vi "ma_sml_Default Center and Span.vi"(0 "fs":dbl=1024.0 format="%.2f", 1 "effective band specification":cluster{"fl (vs. fs)":dbl, "fh (vs. fs)":dbl}={"fl (vs. fs)"=0.0, "fh (vs. fs)"=0.5} {"fh (vs. fs)" format="%.2f"; "fl (vs. fs)" format="%.2f"}, 2 "input signal type":enum16{"real", "complex modulated"}(ring)) -> (3 "f center":dbl=1024.0 format="%.2f", 4 "f upper":dbl=1024.0 format="%.2f", 5 "f lower":dbl=1024.0 format="%.2f", 6 "max span":dbl=1024.0 format="%.2f")   [LabVIEW 2020, in "NI_MAPro.lvlib"]
uses:
  NI_MAPro.lvlib
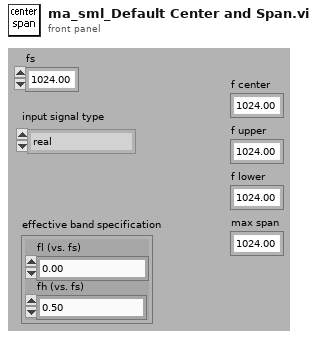
[diagram p1: front panel]
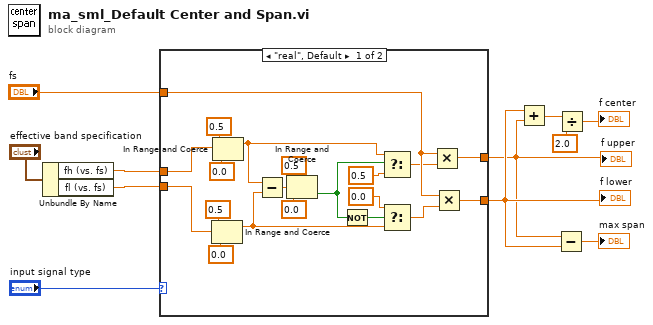
[diagram p0: block diagram]
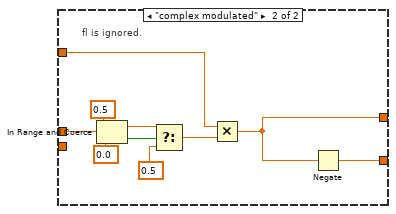
[diagram p2: hidden frame]
diagram:
  n1 = Unbundle By Name("effective band specification") -> ("fh (vs. fs)"=w4:dbl, "fl (vs. fs)"=w5:dbl)
  n2 = case shown="\"real\", Default" "input signal type" {
    tunnel: "fs" -> [w31 w32]
    tunnel: [w30 w34] -> w8
    tunnel: [w29 w33] -> w7
    tunnel: w5 -> [w28 _]
    tunnel: w4 -> [w27 w39]
    frame "real", Default {
      n3 = In Range and Coerce(upper limit=0.5, x=w28, lower limit=0.0) -> (coerced(x)=w16:dbl)  [unwired: 1 out]
      n4 = In Range and Coerce(upper limit=0.5, x=w27, lower limit=0.0) -> (coerced(x)=w19:dbl)  [unwired: 1 out]
      n5 = Subtract(x=w19, y=w16) -> (x-y=w22:dbl)
      n6 = In Range and Coerce(upper limit=0.5 ("x"), x=w22, lower limit=0.0) -> (In Range?=w17:bool)  [unwired: 1 out]
      n7 = Not(x=w17) -> (.not. x?=w15:bool)
      n8 = Select(t=w19, s=w17, f=0.5) -> (s? t:f=w12:dbl)
      n9 = Select(t=0.0, s=w15, f=w16) -> (s? t:f=w13:dbl)
      n10 = Multiply(x=w31, y=w12) -> (x*y=w29:dbl)
      n11 = Multiply(x=w31, y=w13) -> (x*y=w30:dbl)
    }
    frame "complex modulated" {
      # "fl is ignored."
      n12 = In Range and Coerce(upper limit=0.5, x=w39, lower limit=0.0) -> (coerced(x)=w37:dbl, In Range?=w38:bool)
      n13 = Select(t=w37, s=w38, f=0.5) -> (s? t:f=w35:dbl)
      n14 = Multiply(x=w32, y=w35) -> (x*y=w33:dbl)
      n15 = Negate(x=w33) -> (-x=w34:dbl)
    }
  }
  "f upper" <- w7
  "f lower" <- w8
  n16 = Add(x=w8, y=w7) -> (x+y=w3:dbl)
  n17 = Subtract(x=w7, y=w8) -> (x-y=→"max span":dbl)
  n18 = Divide(x=w3, y=2.0) -> (x/y=→"f center":dbl)
